vi "Updater Build New PI File.vi"(8 "error in (no error)":errorcluster, 9 "Channel Name":string, 10 "Source Run ID":string, 11 "Source File":path) -> (0 "error out":errorcluster)   [LabVIEW 2011]
panel:
  out "New Path":path
  out "error out New":errorcluster
  out "error out Source":errorcluster
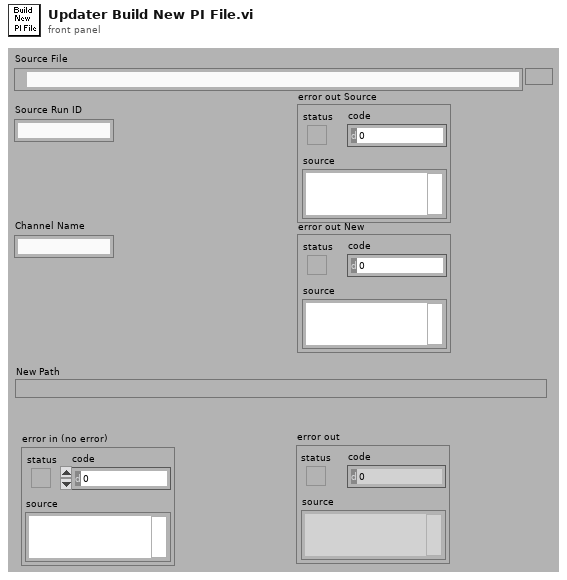
[diagram p1: front panel]
types:
  T1 = enum16{"open", "open or create", "create or replace", "create", "open (read-only)"}
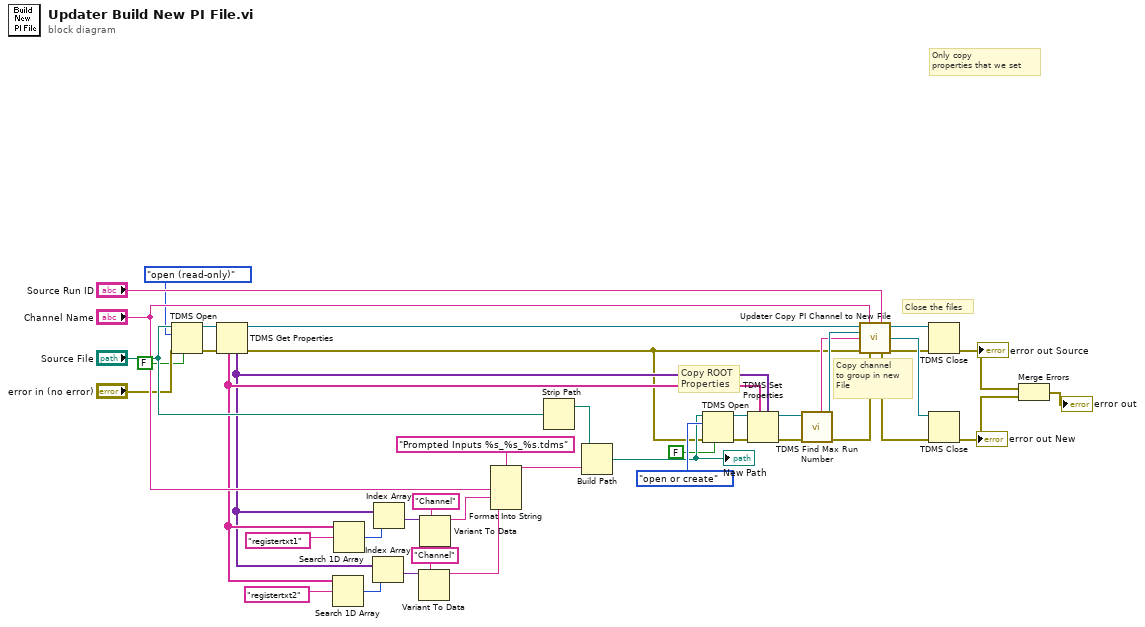
[diagram p0: block diagram]
diagram:
  # "Copy channel\nto group in new\nFile"
  # "Close the files"
  # "Copy ROOT\nProperties"
  # "Only copy \nproperties that we set"
  n1 = TDMS Open(6:FALSE ("disable buffering (T)"), 8:"error in (no error)", 10:T1."open (read-only)" ("operation (0:open)"), 11:"Source File") -> (0:w30:errorcluster, 3:w31:refnum<k34>)  [unwired: 2 in]
  n2 = TDMS Get Properties(8:w30, 11:w31) -> (0:w3:errorcluster, 3:w27:refnum<k34>, 4:w8:variant[], 6:w9:string[])  [unwired: 6 out]
  n3 = Search 1D Array(1D array=w9, element="registertxt2") -> (index of element=w11:i32)  [unwired: 1 out]
  n4 = Search 1D Array(1D array=w9, element="registertxt1") -> (index of element=w16:i32)  [unwired: 1 out]
  n5 = Index Array(array=w8, index=w11) -> (element=w12:variant)
  n6 = Index Array(array=w8, index=w16) -> (element=w15:variant)
  n7 = Variant To Data(type="Channel", Variant=w12) -> (data=w6:string)  [unwired: 1 in, 1 out]
  n8 = Variant To Data(type="Channel", Variant=w15) -> (data=w7:string)  [unwired: 1 in, 1 out]
  n9 = Format Into String(format string="Prompted Inputs %s_%s_%s.tdms", "Channel Name", w7, w6) -> (resulting string=w41:string)  [unwired: 2 in, 1 out]
  n10 = Strip Path(path="Source File") -> (stripped path=w40:path)  [unwired: 1 out]
  n11 = Build Path(base path=w40, name or relative path=w41) -> (appended path=w5:path)
  "New Path" <- w5
  n12 = TDMS Open(6:FALSE ("disable buffering (T)"), 8:w3, 10:T1."open or create" ("operation (0:open)"), 11:w5) -> (0:w28:errorcluster, 3:w29:refnum<k34>)  [unwired: 2 in]
  n13 = TDMS Set Properties(5:w8, 7:w9, 8:w28, 11:w29) -> (0:w22:errorcluster, 3:w21:refnum<k34>)  [unwired: 4 out]
  n14 = call "TDMS Find Max Run Number.vi"("error in (no error)"=w22, "tdms file"=w21) -> ("error out"=w18:errorcluster, "tdms file out"=w20:refnum<k34>, "Next Run ID"=w19:string)  [unwired: 7 out]
  n15 = call "Updater Copy PI Channel to New File.vi"("Source tdms file in"=w27, "Channel Name"="Channel Name", "Source Run ID"="Source Run ID", "New tdms file in"=w20, "New Run #"=w19, "error out 4"=w3, "error out"=w18) -> ("tdms file out 2"=w24:refnum<k34>, "tdms file out 3"=w26:refnum<k34>, "error out 3"=w25:errorcluster, "error out 2"=w23:errorcluster)  [unwired: 1 in, 4 out]
  n16 = TDMS Close(8:w23, 11:w24) -> (0:w36:errorcluster)  [unwired: 1 out]
  "error out Source" <- w36
  n17 = TDMS Close(8:w25, 11:w26) -> (0:w35:errorcluster)  [unwired: 1 out]
  "error out New" <- w35
  n18 = Merge Errors(w36, w35) -> (→"error out":errorcluster)
